vi "Update Tool Cfg from Local XML File.vi"(8 "error in (no error)":errorcluster, 11 "Cfg File Path":path=path "/home/lvuser/natinst/QCX Tool Cfg.xml") -> (0 "error out":errorcluster, 3 "Tool Config Cluster":T1={"Tool Type"=0, "Tool SN"=0, "Tool Block"={"Encoder Size"=0, "Encoder Scale"=0, "Encoder Offset"=0, "MaxEncoder"=0, "MinEncoder"=0, "Start Delay"=0.0, "Tool Face Ref"=0.0}, "Motor Block"={"MinMotor Speed"=0, "MaxMotor Speed"=0, "Homing Speed"=90, "Jog Speed"=90, "Inspect Speed"=90, "VBlk Speed"=90, "CleaningPos"=0, "Safe Zone"=0, "Has Motor"=FALSE, "Use Home Index"=FALSE}, "Verification Block"={"Angle"=90.0, "FlankLength1"=0.0, "FlankLength2"=0.0, "Location"=0.0, "Serial Number"=0}, "Probe Block"={"nProbes"=0, "Probe Param Array"=[]}} {"Probe Block"."Probe Param Array"."Sensor Block"."SensorCfgParams Array"."CalibrCoefArray" format="%#.12g"})   [LabVIEW 2015, in "Tool Cfg.lvlib"]
uses:
  Tool Cfg.lvlib
  _Configuration Cluster_v3--typedef.ctl
  _Tool Block Cluster_v3--typedef.ctl
  _Motor Block Cluster_v2--typedef.ctl
  _Verification Blk Cluster--typedef.ctl
  _ProbeConfigParams Cluster--typedef.ctl
  _Sensor Block Cluster--typedef.ctl
  _SensorConfigParams Cluster--typedef.ctl
  _Configuration Cluster_v1--typedef.ctl
  _Tool Block Cluster--typedef.ctl
  _Motor Block Cluster_v1--typedef.ctl
  _Probe Block Cluster--typedef.ctl
  _Configuration Cluster_v2--typedef.ctl
  <vilib>/Utility/xml.llb/Read From XML File(array).vi
  ConfigGLOB.vi
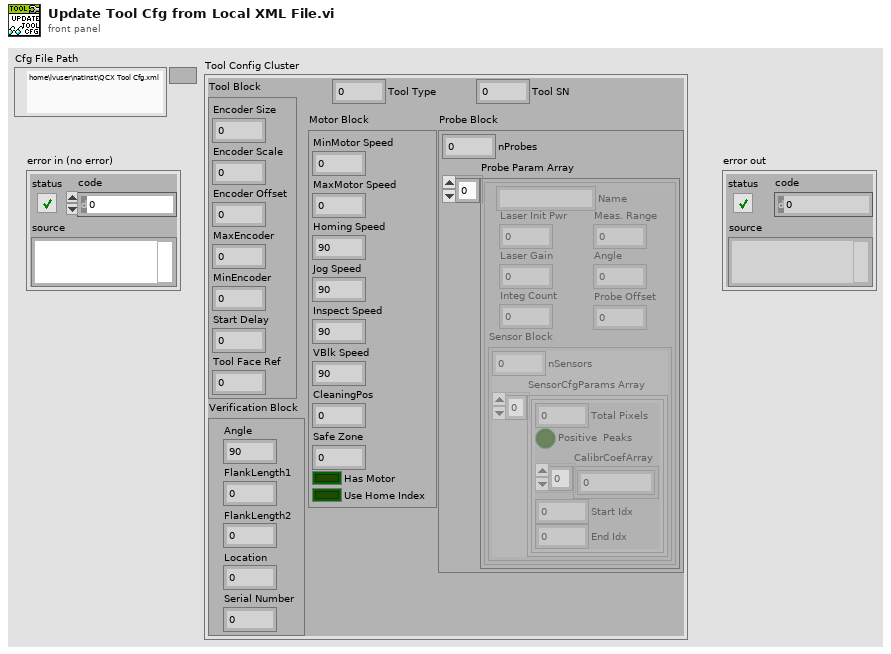
[diagram p1: front panel]
types:
  T1 = typedef "Tool Cfg.lvlib/_Configuration Cluster_v3--typedef.ctl" = cluster{"Tool Type":u16, "Tool SN":u16, "Tool Block":T2, "Motor Block":T3, "Verification Block":T4, "Probe Block":cluster{"nProbes":u16, "Probe Param Array":T5[]}}
  T2 = typedef "Tool Cfg.lvlib/_Tool Block Cluster_v3--typedef.ctl" = cluster{"Encoder Size":u16, "Encoder Scale":u32, "Encoder Offset":i32, "MaxEncoder":i32, "MinEncoder":i32, "Start Delay":sgl, "Tool Face Ref":sgl}
  T3 = typedef "Tool Cfg.lvlib/_Motor Block Cluster_v2--typedef.ctl" = cluster{"MinMotor Speed":u16, "MaxMotor Speed":u16, "Homing Speed":u16, "Jog Speed":u16, "Inspect Speed":u16, "VBlk Speed":u16, "CleaningPos":i32, "Safe Zone":i32, "Has Motor":bool, "Use Home Index":bool}
  T4 = typedef "Tool Cfg.lvlib/_Verification Blk Cluster--typedef.ctl" = cluster{"Angle":sgl, "FlankLength1":sgl, "FlankLength2":sgl, "Location":sgl, "Serial Number":u16}
  T5 = typedef "Tool Cfg.lvlib/_ProbeConfigParams Cluster--typedef.ctl" = cluster{"Name":string, "Laser Init Pwr":u16, "Laser Gain":u8, "Integ Count":u16, "Meas. Range":sgl, "Angle":sgl, "Probe Offset":sgl, "Sensor Block":T6}
  T6 = typedef "Tool Cfg.lvlib/_Sensor Block Cluster--typedef.ctl" = cluster{"nSensors":u16, "SensorCfgParams Array":T7[]}
  T7 = typedef "Tool Cfg.lvlib/_SensorConfigParams Cluster--typedef.ctl" = cluster{"Total Pixels":u16, "Positive  Peaks":bool, "CalibrCoefArray":dbl[], "Start Idx":u16, "End Idx":u16}
  T8 = typedef "Tool Cfg.lvlib/_Configuration Cluster_v1--typedef.ctl" = cluster{"Tool Type":u16, "Tool SN":u16, "Tool Block":T9, "Motor Block":T10, "Verification Block":T4, "Probe Block":T11}
  T9 = typedef "Tool Cfg.lvlib/_Tool Block Cluster--typedef.ctl" = cluster{"Encoder Size":u16, "Encoder Scale":u32, "Encoder Offset":i32, "MaxEncoder":i32, "MinEncoder":i32, "Start Delay":sgl}
  T10 = typedef "Tool Cfg.lvlib/_Motor Block Cluster_v1--typedef.ctl" = cluster{"MinMotor Speed":u16, "MaxMotor Speed":u16, "Homing Speed":u16, "Jog Speed":u16, "Inspect Speed":u16, "VBlk Speed":u16, "CleaningPos":i32, "Has Motor":bool, "Use Home Index":bool}
  T11 = typedef "Tool Cfg.lvlib/_Probe Block Cluster--typedef.ctl" = cluster{"nProbes":u16, "Probe Param Array":T5[]}
  T12 = typedef "Tool Cfg.lvlib/_Configuration Cluster_v2--typedef.ctl" = cluster{"Tool Type":u16, "Tool SN":u16, "Tool Block":T9, "Motor Block":T3, "Verification Block":T4, "Probe Block":T11}
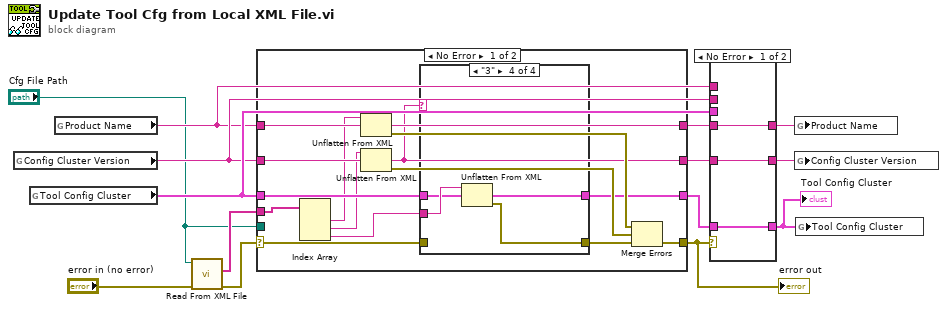
[diagram p0: block diagram]
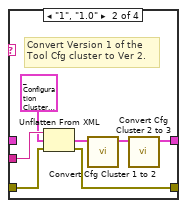
[diagram p3: hidden frame]
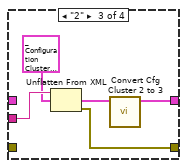
[diagram p4: hidden frame]
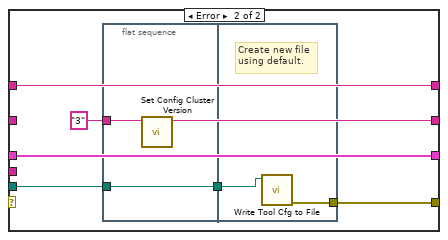
[diagram p5: hidden frame]
diagram:
  n1 = global read "ConfigGLOB.vi" "Config Cluster Version"() -> (w6:string)
  n2 = global read "ConfigGLOB.vi" "Tool Config Cluster"() -> (w7:T1)
  n3 = global read "ConfigGLOB.vi" "Product Name"() -> (w5:string)
  n4 = call-poly <vilib>:"Read From XML File.vi"("error in (no error)"="error in (no error)", "XML File Path"="Cfg File Path") -> ("error out"=w14:errorcluster, "XML Elements"=w13:string[])  [unwired: 7 in, 1 out]
  n5 = case shown="No Error" w14 {
    selector: w14 -> [w18 _]
    tunnel: w13 -> [w21 _]
    tunnel: w7 -> [w28 w53]
    tunnel: [w17 w53] -> w10
    tunnel: [w27 w51] -> w11
    tunnel: w6 -> [w29 _]
    tunnel: [w15 w48] -> w9
    tunnel: w5 -> [w24 w52]
    tunnel: [w22 w52] -> w3
    tunnel: "Cfg File Path" -> [_ w50]
    frame No Error {
      n6 = Index Array(array=w21) -> (element #1=w23:string, element #2=w20:string, element #3=w19:string)  [unwired: 3 in]
      n7 = Unflatten From XML(xml string=w23, type=w24) -> (value=w22:string, error out=w25:errorcluster)  [unwired: 1 in]
      n8 = Unflatten From XML(xml string=w20, type=w29) -> (value=w15:string, error out=w26:errorcluster)  [unwired: 1 in]
      n9 = case shown="\"3\"" w15 {
        tunnel: w28 -> [w31 _ _ w44]
        tunnel: w19 -> [_ w38 w42 w46]
        tunnel: w18 -> [w30 w37 _ _]
        tunnel: [w31 w32 w40 w45] -> w17
        tunnel: [w30 w34 w43 w47] -> w16
        frame Default {
        }
        frame "1", "1.0" {
          # "Convert Version 1 of the Tool Cfg cluster to Ver 2."
          n10 = Unflatten From XML(xml string=w38, type=T8 {"Tool Type"=0, "Tool SN"=0, "Tool Block"={"Encoder Size"=0, "Encoder Scale"=0, "Encoder Offset"=0, "MaxEncoder"=0, "MinEncoder"=0, "Start Delay"=0.0}, "Motor Block"={"MinMotor Speed"=0, "MaxMotor Speed"=0, "Homing Speed"=90, "Jog Speed"=90, "Inspect Speed"=90, "VBlk Speed"=90, "CleaningPos"=0, "Has Motor"=FALSE, "Use Home Index"=FALSE}, "Verification Block"={"Angle"=90.0, "FlankLength1"=0.0, "FlankLength2"=0.0, "Location"=0.0, "Serial Number"=0}, "Probe Block"={"nProbes"=0, "Probe Param Array"=[]}} ("_Tool Config Cluster_v1--typedef"), error in (no error)=w37) -> (value=w35:T8, error out=w34:errorcluster)
          n11 = call "Convert Cfg Cluster 1 to 2.vi"("Tool Config Cluster_v1"=w35) -> ("Tool Config Cluster_v2"=w33:T12)  [unwired: 10 in]
          n12 = call "Convert Cfg Cluster 2 to 3.vi"("Tool Config Cluster_v2"=w33) -> ("Tool Config Cluster_v3"=w32:T1)  [unwired: 10 in]
        }
        frame "2" {
          n13 = Unflatten From XML(xml string=w42, type=T12 {"Tool Type"=0, "Tool SN"=0, "Tool Block"={"Encoder Size"=0, "Encoder Scale"=0, "Encoder Offset"=0, "MaxEncoder"=0, "MinEncoder"=0, "Start Delay"=0.0}, "Motor Block"={"MinMotor Speed"=0, "MaxMotor Speed"=0, "Homing Speed"=90, "Jog Speed"=90, "Inspect Speed"=90, "VBlk Speed"=90, "CleaningPos"=0, "Safe Zone"=0, "Has Motor"=FALSE, "Use Home Index"=FALSE}, "Verification Block"={"Angle"=90.0, "FlankLength1"=0.0, "FlankLength2"=0.0, "Location"=0.0, "Serial Number"=0}, "Probe Block"={"nProbes"=0, "Probe Param Array"=[]}} ("_Tool Config Cluster_v2--typedef")) -> (value=w41:T12, error out=w43:errorcluster)  [unwired: 1 in]
          n14 = call "Convert Cfg Cluster 2 to 3.vi"("Tool Config Cluster_v2"=w41) -> ("Tool Config Cluster_v3"=w40:T1)  [unwired: 10 in]
        }
        frame "3" {
          n15 = Unflatten From XML(xml string=w46, type=w44) -> (value=w45:T1, error out=w47:errorcluster)  [unwired: 1 in]
        }
      }
      n16 = Merge Errors(w25, w26, w16) -> (w27:errorcluster)
    }
    frame Error {
      w48 = "3" ("Config Cluster Version")
      n17 = flat-sequence {
        tunnel: w50 -> [w55]
        tunnel: [w55] -> w49
        tunnel: w48 -> [w54]
        tunnel: [w57] -> w51
        tunnel: w49 -> [w56]
        frame #0 {
          n18 = call "Set Config Cluster Version.vi"("Config Cluster Version"=w54) -> ()  [unwired: 11 in]
        }
        frame #1 {
          # "Create new file\nusing default."
          n19 = call "Write Tool Cfg to File.vi"("Cfg File Path"=w56) -> ("error out"=w57:errorcluster)  [unwired: 10 in]
        }
      }
    }
  }
  "error out" <- w11
  n20 = case shown="No Error" w11 {
    tunnel: w10 -> [w60 _]
    tunnel: [w60 w63] -> w1
    tunnel: w9 -> [w59 _]
    tunnel: [w59 w62] -> w8
    tunnel: w7 -> [_ w63]
    tunnel: w6 -> [_ w62]
    tunnel: w5 -> [_ w61]
    tunnel: [w58 w61] -> w4
    tunnel: w3 -> [w58 _]
    frame No Error {
    }
    frame Error {
    }
  }
  "Tool Config Cluster" <- w1
  n21 = global write "ConfigGLOB.vi" "Product Name"(w4) -> ()
  n22 = global write "ConfigGLOB.vi" "Config Cluster Version"(w8) -> ()
  n23 = global write "ConfigGLOB.vi" "Tool Config Cluster"(w1) -> ()
